vi "Read lst.vi"(8 "error in (no error)":errorcluster, 11 "CurrentTimes in":refnum<class "CurrentTimes.lvclass">) -> (0 "error out":errorcluster, 2 "ClockTimes.lvclass":refnum<class "ClockTimes.lvclass">, 3 "CurrentTimes out":refnum<class "CurrentTimes.lvclass">)   [LabVIEW 2014, in "TCSDataDefinitions.lvlib" / "TCSPublicStatus.lvlib" / "CurrentTimes.lvlib" / "CurrentTimes.lvclass"]
uses:
  CurrentTimes.lvclass
  ClockTimes/ClockTimes.lvclass
  CurrentTimes.lvclass/CurrentTimes.ctl
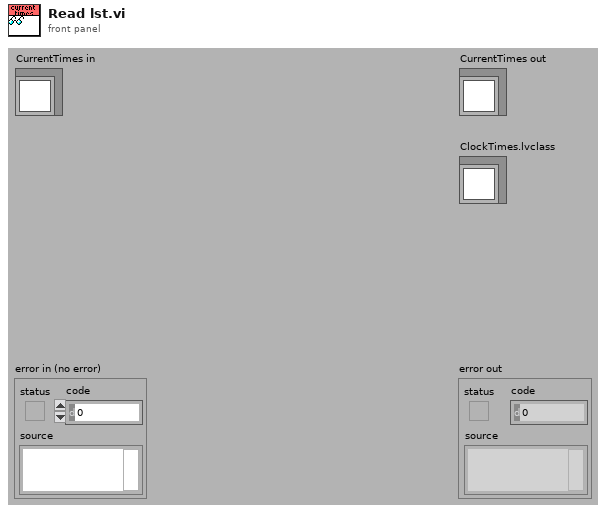
[diagram p1: front panel]
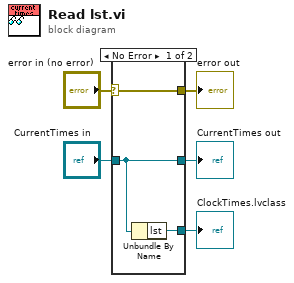
[diagram p0: block diagram]
diagram:
  n1 = case shown="No Error" "error in (no error)" {
    selector: "error in (no error)" -> [w8 w9]
    tunnel: [w8 w9] -> w4
    tunnel: [w7 w10] -> w2
    tunnel: "CurrentTimes in" -> [w7 w10]
    tunnel: [w6 _] -> w1
    frame No Error {
      n2 = Unbundle By Name(w7) -> ("lst"=w6:refnum<class "ClockTimes.lvclass">)
    }
    frame Error {
    }
  }
  "error out" <- w4
  "CurrentTimes out" <- w2
  "ClockTimes.lvclass" <- w1
